vi "matrix pgm.vi"(6 "matrixSize":i32, 7 "normalize":i32, 9 "gamma":i32, 10 "matrix":dbl[](array[numeric])=array[4097 elements], 11 "path":string) -> (2 "matrix out":dbl[](array[numeric]))   [LabVIEW 2012, in "LightPipes.lvlib"]
doc: "__declspec(dllexport) void matrix_pgm(const char *path, double matrix[], int gamma, int normalize, int matrixSize);"
uses:
  LightPipes.lvlib
  VS Project/Debug/Lightpipes.dll
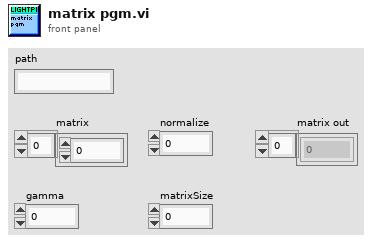
[diagram p1: front panel]
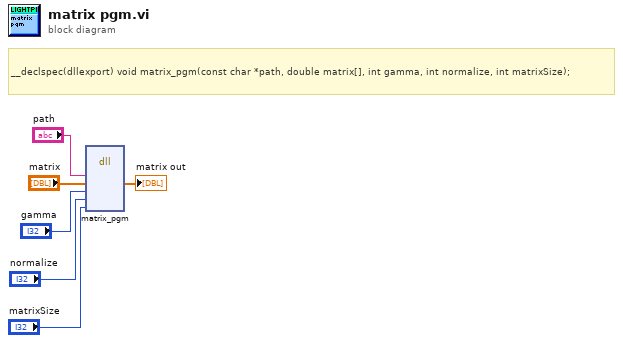
[diagram p0: block diagram]
diagram:
  # "__declspec(dllexport) void matrix_pgm(const char *path, double matrix[], int gamma, int normalize, int matrixSize);"
  n1 = dll-call lib="C:/Users/Tri/Documents/Lightpipes/VS Project/Debug/Lightpipes.*" fn="matrix_pgm"("path"="path", "matrix"="matrix", "gamma"="gamma", "normalize"="normalize", "matrixSize"="matrixSize") -> ("matrix"=→"matrix out":dbl[])  [unwired: 8 in, 2 out]
